vi "Get Pos Impl.vi"(8 "error in (no error)":errorcluster, 11 "Ludl Stage in":refnum<class "Ludl Stage.lvclass">) -> (0 "error out":errorcluster, 2 "Stage Position":T1, 3 "Ludl Stage out":refnum<class "Ludl Stage.lvclass">)   [LabVIEW 2023, in "Ludl Stage.lvlib" / "Ludl Stage.lvclass"]
uses:
  Resources/Type Defs/Stage Position.ctl
  Ludl Stage.lvclass
  Ludl Stage.lvclass/Ludl Stage.ctl
  Stage Controller/Stage Controller.lvlib
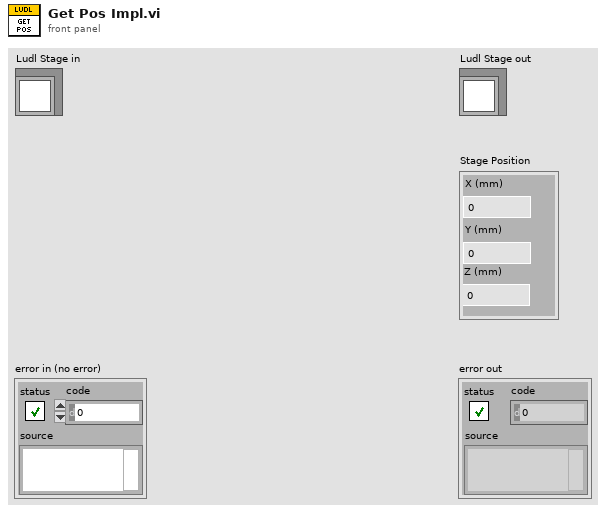
[diagram p1: front panel]
types:
  T1 = typedef "Stage Position.ctl" = cluster{"X (mm)":dbl, "Y (mm)":dbl, "Z (mm)":dbl}
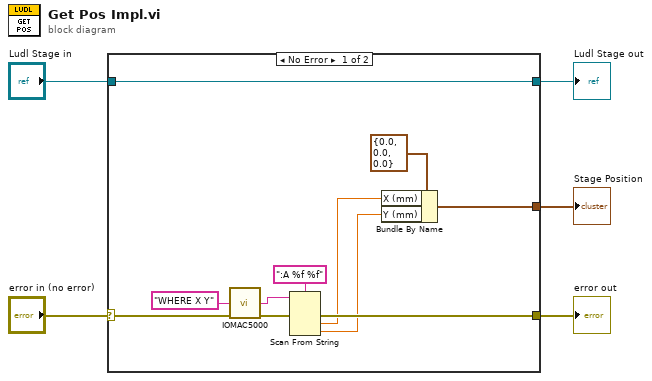
[diagram p0: block diagram]
diagram:
  n1 = case shown="No Error" "error in (no error)" {
    selector: "error in (no error)" -> [w6 w17]
    tunnel: [w12 w17] -> w5
    tunnel: [w10 _] -> w4
    tunnel: "Ludl Stage in" -> [w7 w18]
    tunnel: [w7 w18] -> w2
    frame No Error {
      n2 = call "IOMAC5000.vi"("Command (to ctlr)"="WHERE X Y" ("format string"), "error in"=w6) -> ("Raw Response"=w15:string, "error out"=w13:errorcluster)  [unwired: 10 in, 2 out]
      n3 = Scan From String(format string=":A %f %f", input string=w15, error in=w13) -> (error out=w12:errorcluster, output 1=w9:dbl, output 2=w8:dbl)  [unwired: 3 in, 2 out]
      n4 = Bundle By Name(cluster=T1 {"X (mm)"=0.0, "Y (mm)"=0.0, "Z (mm)"=0.0} ("Stage Position 2"), "X (mm)"=w9, "Y (mm)"=w8) -> (w10:T1)
    }
    frame Error {
    }
  }
  "error out" <- w5
  "Ludl Stage out" <- w2
  "Stage Position" <- w4
